vi "VendingMachine - Gavin Branyon.vi"() -> ()   [LabVIEW 2019]
panel:
  in  "Product 3":bool
  in  "Product 2":bool
  in  "Product 1":bool
  in  "stop":bool
  out "Deposited":i32
  in  "Quarter":bool
  in  "Dime":bool
  in  "Nickel":bool
  # "Gavin Branyon\nSoda Dispensor\n3/18/2024"
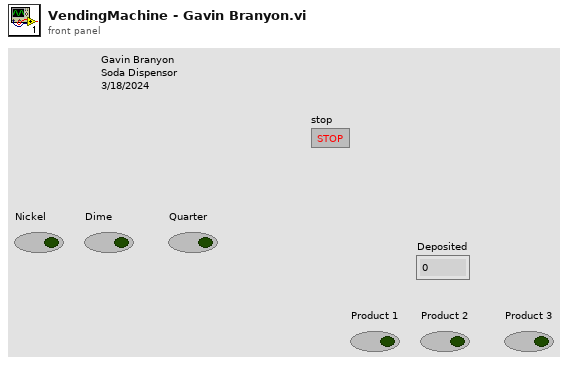
[diagram p1: front panel]
types:
  T1 = enum16{"Idle", "Adding Coins", "Select Product", "Dispense Product", "Return Change"}
  T2 = enum16{"Idle", "Adding Coins", "Select Product", "Dispense Product"}
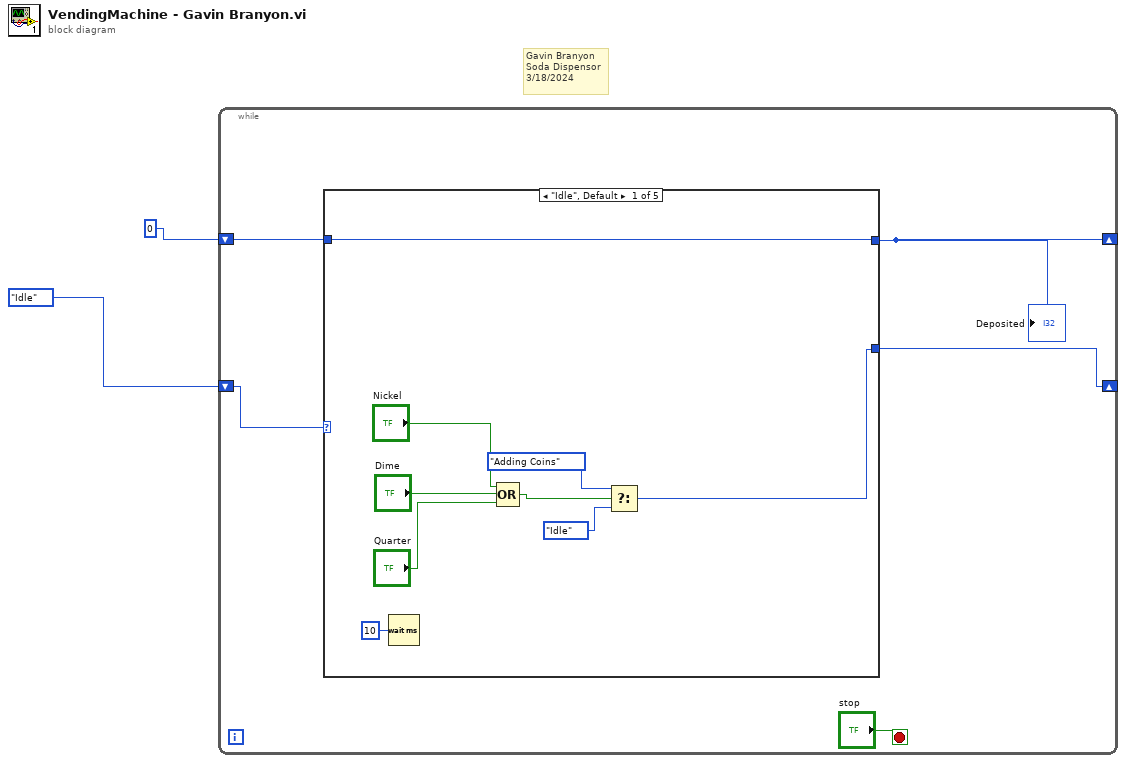
[diagram p0: block diagram]
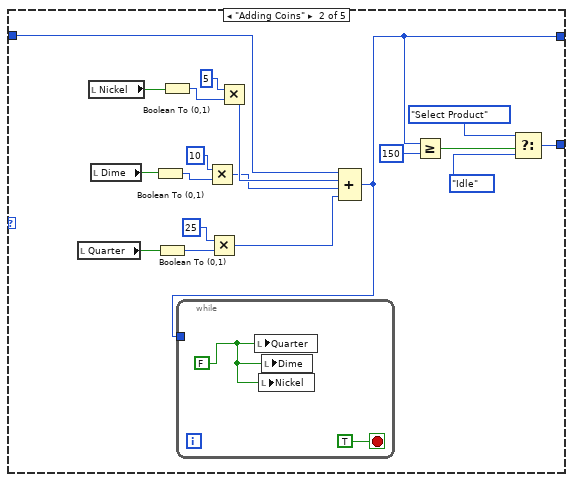
[diagram p2: hidden frame]
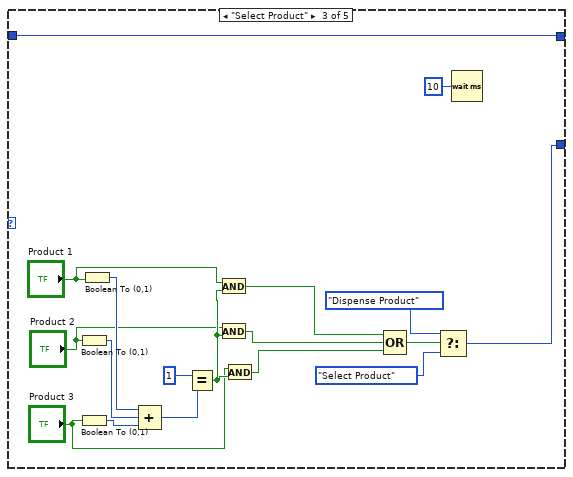
[diagram p3: hidden frame]
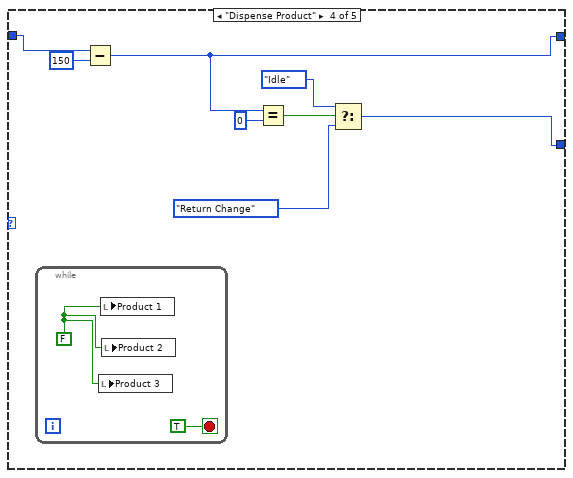
[diagram p4: hidden frame]
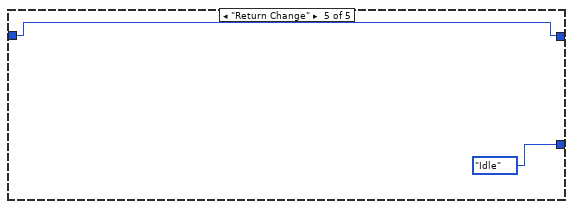
[diagram p5: hidden frame]
diagram:
  # "Gavin Branyon\nSoda Dispensor\n3/18/2024"
  n1 = while {
    shift-right: [w3] -> _
    shift-left: T1."Idle" ("Enum") -> [w7]
    shift-right: [w5] -> _
    shift-left: 0 -> [w6]
    stop <- "stop" stop-if-true
    n2 = case shown="\"Idle\", Default" w7 {
      tunnel: w6 -> [w8 w26 w52 w63 w66]
      tunnel: [w8 w22 w52 w61 w66] -> w5
      tunnel: [w9 w17 w53 w58 T2."Idle" ("Enum")] -> w3
      frame "Idle", Default {
        n3 = Wait (ms)(milliseconds to wait=u32 10) -> ()  [unwired: 1 out]
        n4 = Compound Arithmetic op=OR("Nickel", "Dime", "Quarter") -> (w13:bool)
        n5 = Select(t=T2."Adding Coins" ("Enum"), s=w13, f=T2."Idle" ("Enum")) -> (s? t:f=w9:T2)
      }
      frame "Adding Coins" {
        n6 = local read "Quarter"() -> (w34:bool)
        n7 = local read "Nickel"() -> (w35:bool)
        n8 = local read "Dime"() -> (w33:bool)
        n9 = Boolean To (0,1)(Boolean=w33) -> (0, 1=w31:i16)
        n10 = Boolean To (0,1)(Boolean=w34) -> (0, 1=w32:i16)
        n11 = Boolean To (0,1)(Boolean=w35) -> (0, 1=w30:i16)
        n12 = Multiply(x=i16 10, y=w31) -> (x*y=w24:i16)
        n13 = Multiply(x=i16 25, y=w32) -> (x*y=w23:i16)
        n14 = Multiply(x=i16 5, y=w30) -> (x*y=w25:i16)
        n15 = Compound Arithmetic op=ADD(w26, w25, w24, w23) -> (w22:i32)
        n16 = while {
          tunnel: w22 -> [_]
          stop <- TRUE stop-if-true
          w36 = FALSE
          n17 = local write "Quarter"(w36) -> ()
          n18 = local write "Nickel"(w36) -> ()
          n19 = local write "Dime"(w36) -> ()
        }
        n20 = Greater Or Equal?(x=w22, y=150) -> (x >= y?=w20:bool)
        n21 = Select(t=T2."Select Product" ("Enum"), s=w20, f=T2."Idle" ("Enum")) -> (s? t:f=w17:T2)
      }
      frame "Select Product" {
        n22 = Boolean To (0,1)(Boolean="Product 2") -> (0, 1=w49:i16)
        n23 = Boolean To (0,1)(Boolean="Product 3") -> (0, 1=w48:i16)
        n24 = Boolean To (0,1)(Boolean="Product 1") -> (0, 1=w50:i16)
        n25 = Compound Arithmetic op=ADD(w50, w49, w48) -> (w47:i16)
        n26 = Equal?(x=i16 1, y=w47) -> (x = y?=w46:bool)
        n27 = And(x="Product 1", y=w46) -> (x .and. y?=w42:bool)
        n28 = And(x="Product 2", y=w46) -> (x .and. y?=w41:bool)
        n29 = And(x="Product 3", y=w46) -> (x .and. y?=w40:bool)
        n30 = Compound Arithmetic op=OR(w42, w41, w40) -> (w39:bool)
        n31 = Select(t=T2."Dispense Product" ("Enum"), s=w39, f=T2."Select Product" ("Enum")) -> (s? t:f=w53:T2)
        n32 = Wait (ms)(milliseconds to wait=u32 10) -> ()  [unwired: 1 out]
      }
      frame "Dispense Product" {
        n33 = while {
          stop <- TRUE stop-if-true
          w65 = FALSE ("Product 1")
          n34 = local write "Product 3"(w65) -> ()
          n35 = local write "Product 1"(w65) -> ()
          n36 = local write "Product 2"(w65) -> ()
        }
        n37 = Subtract(x=w63, y=150) -> (x-y=w61:i32)
        n38 = Equal?(x=w61, y=0) -> (x = y?=w59:bool)
        n39 = Select(t=T2."Idle" ("Enum"), s=w59, f=T1."Return Change" ("Enum")) -> (s? t:f=w58:T1)
      }
      frame "Return Change" {
      }
    }
    "Deposited" <- w5
  }
